vi "Add Note.vi"(6 "timeout (ms)":i32=-1, 8 "error in (no error)":errorcluster, 10 "Note":string, 11 "FlexLogger_gRPCAPI in":refnum<class "FlexLogger_gRPC.lvclass">) -> (0 "error out":errorcluster, 3 "FlexLogger_gRPCAPI out":refnum<class "FlexLogger_gRPC.lvclass">)   [LabVIEW 2020, in "FlexLogger_gRPC.lvlib" / "FlexLogger_gRPC.lvclass"]
doc: "Adds a note to the log file. Notes can only be added while the test session is running."
uses:
  FlexLogger_gRPC.lvclass
  FlexLogger_client/RPC Messages/flexlogger_AddNoteRequest.ctl
  FlexLogger_gRPC.lvclass/FlexLogger_gRPC.ctl
  FlexLogger_client/FlexLogger_client.lvlib
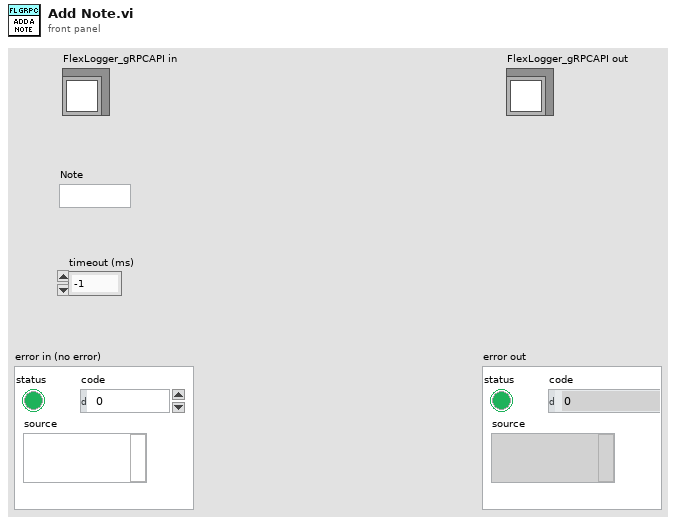
[diagram p1: front panel]
types:
  T1 = typedef "FlexLogger_client.lvlib/flexlogger_AddNoteRequest.ctl" = cluster{"note":string}
  T2 = typedef "grpc-lvsupport-release.lvlib/grpcId.ctl" = u64
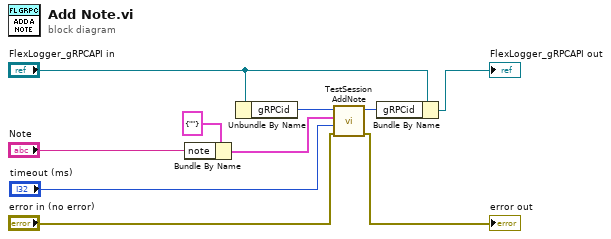
[diagram p0: block diagram]
diagram:
  n1 = Bundle By Name(cluster=T1 {"note"=""} ("Request Data"), "note"="Note") -> (w8:T1)
  n2 = Unbundle By Name("FlexLogger_gRPCAPI in") -> ("gRPCid"=w7:T2)
  n3 = call "TestSession AddNote.vi"("error in"="error in (no error)", "timeout (ms)"="timeout (ms)", "Request Data"=w8, "gRPC ID"=w7) -> ("error out"=→"error out":errorcluster, "gRPC ID out"=w5:T2)  [unwired: 5 in, 1 out]
  n4 = Bundle By Name(cluster="FlexLogger_gRPCAPI in", "gRPCid"=w5) -> (→"FlexLogger_gRPCAPI out":refnum<class "FlexLogger_gRPC.lvclass">)
